vi "Amaster.vi"(8 "ErrorIn":errorcluster, 11 "AQueuesIn":T1) -> (0 "ErrorOut":errorcluster, 3 "AQueuesOut":T1)   [LabVIEW 2019]
uses:
  utilities/AQueues.ctl
  AmasterVIs/ACommand.ctl
  analyzeAccelerationDataVIs/AccelerationDataFrames.ctl
  analyzeAccelerationDataVIs/AnalyzedVibrationsData.ctl
  analyzeAccelerationDataVIs/calculateFaultIndicatorsVIs/FaultDetections.ctl
  analyzeAccelerationDataVIs/calculateFaultIndicatorsVIs/ParameterFaultDetection.ctl
  analyzeAccelerationDataVIs/calculateFaultIndicatorsVIs/FaultParameter.ctl
  analyzeAccelerationDataVIs/calculateFaultIndicatorsVIs/FrequencyFaultDetection.ctl
  analyzeAccelerationDataVIs/calculateFaultIndicatorsVIs/OrdersFaultDetection.ctl
  TDMSmanagerVIs/TDMSAnalyzerData.ctl
  TDMSmanagerVIs/TDMSAnalyzerDataType.ctl
  <vilib>/Platform/TimedLoop/XDataNode/timing_clust.ctl
  <vilib>/Platform/TimedLoop/XDataNode/nitl_modes.ctl
  <vilib>/Platform/TimedLoop/XDataNode/wakeup.ctl
  AmasterVIs/ACommandQueuesAction.ctl
  AmasterVIs/AThreads.ctl
  UIVIs/UIOutputFGVAction.ctl
  <vilib>/platform/TimedLoop/XDataNode/XDataNode.xnode
  <vilib>/Platform/TimedLoop/XDataNode/XDNodeRunTimeDep.lvlib
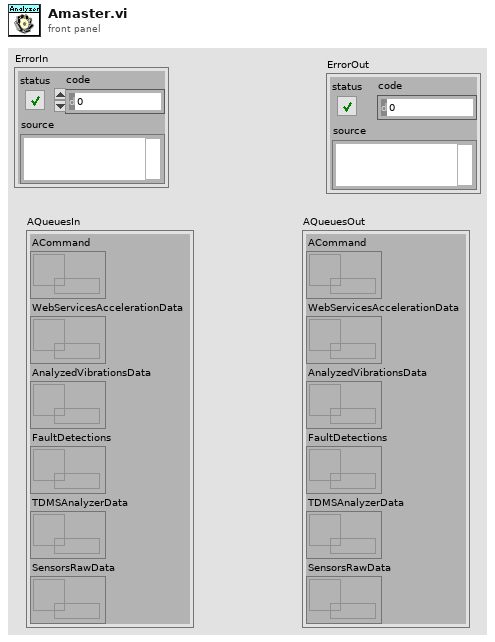
[diagram p1: front panel]
types:
  T1 = typedef "AQueues.ctl" = cluster{"ACommand":refnum<queue>, "WebServicesAccelerationData":refnum<queue>, "AnalyzedVibrationsData":refnum<queue>, "FaultDetections":refnum<queue>, "TDMSAnalyzerData":refnum<queue>, "SensorsRawData":refnum<queue>}
  T2 = typedef "XDNodeRunTimeDep.lvlib/timing_clust.ctl" = cluster{"Expected End [f-1]":u64, "Actual End [f-1]":u64, "Finished Late? [f-1]":bool, "Expected End [i-1]":u64, "Actual End [i-1]":u64, "Finished Late? [i-1]":bool, "Expected Start [i]":u64, "Actual Start [i]":u64, "Expected Start [f]":u64, "Actual Start [f]":u64, "Source Name":string, "Structure Name":string, "Period":i64, "Deadline":i64, "Offset":i64, "Start":i64, "Priority":i32, "Timeout":i32, "Mode":T3, "Wakeup Reason":T4, "Error":errorcluster, "Source Type":string, "Secondary Source Type":string, "Global End Time":u64, "Global Start Time":u64, "Frame Duration":u64, "Iteration Duration":u64, "Assigned CPU":i32, "I/O Scan Engine Mode":u32}
  T3 = typedef "XDNodeRunTimeDep.lvlib/nitl_modes.ctl" = enum32{"No Change", "Process missed periods, maintain original phase", "Discard missed periods, maintain original phase", "Process missed periods, ignore original phase", "Discard missed periods, ignore original phase"}
  T4 = typedef "XDNodeRunTimeDep.lvlib/wakeup.ctl" = enum32{"Normal", "Aborted", "Asynchronous wakeup", "Timing source error", "Timed loop error", "Timeout"}
  T5 = typedef "ACommandQueuesAction.ctl" = enum16{"Initialize", "Set", "Get", "ReleaseAll"}
  T6 = typedef "UIOutputFGVAction.ctl" = enum16{"Read", "Write", "CheckUpdate"}
  T7 = typedef "ACommand.ctl" = enum16{"None", "Start", "Stop", "Restart", "SendFilesData", "DeleteAllData"}
  T8 = typedef "AThreads.ctl" = enum16{"UI", "analyzeAccelerationData", "aquireAccelerationData", "communicateWebServices", "TDMSmanager", "aquireTachoSignal"}
  T9 = typedef "AnalyzerSettings.ctl" = cluster{"Create NS Timeout Code":i32, "Destroy NS Timeout Code":i32, "All threads":T8[], "AnalysisSettings":T10}
  T10 = typedef "AnalysisSettings.ctl" = cluster{"Fault Thresholds":T11, "Analysis series name":string, "Save data analysis?":bool, "Band size":i32, "OrderAnalysis?":bool, "Accelerometer":T13, "fs [Hz]":dbl, "Pulse per revolution":u16}
  T11 = typedef "Thresholds.ctl" = cluster{"Parameters labels":T12[], "Parameters thresholds":dbl[], "Freqs and thresholds":dbl[][], "Orders and thresholds":dbl[][]}
  T12 = typedef "FaultParameter.ctl" = enum16{"Kurtosis", "RMS", "Crest factor"}
  T13 = typedef "Accelerometer.ctl" = enum16{"None", "MPU6050", "MMA7351"}
  T14 = typedef "UIOutput.ctl" = cluster{"Aquiring data":bool, "AnalyzerError":errorcluster, "FIFO overflow":bool, "Analyzing data":bool}
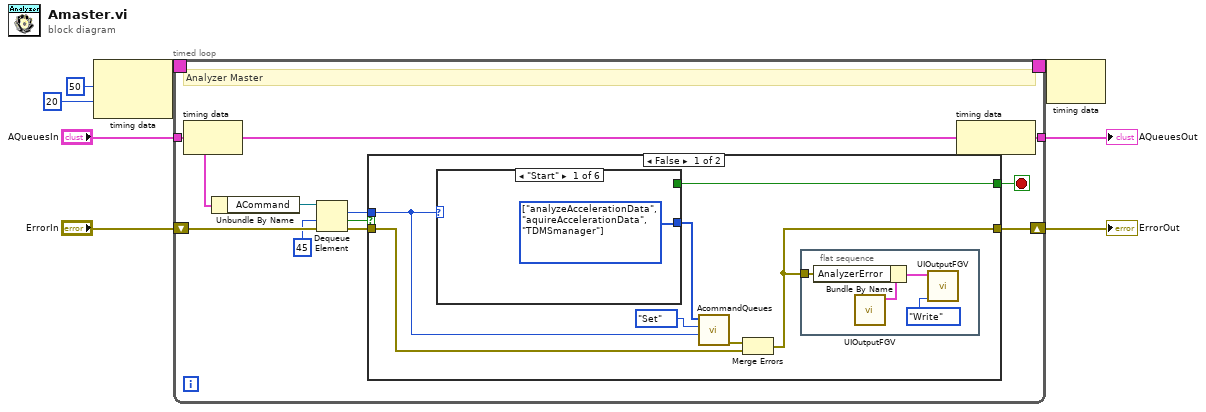
[diagram p0: block diagram]
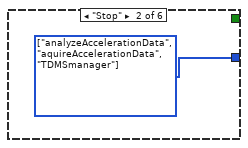
[diagram p2: hidden frame]
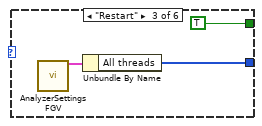
[diagram p3: hidden frame]
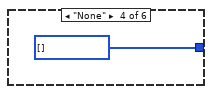
[diagram p4: hidden frame]
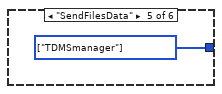
[diagram p5: hidden frame]
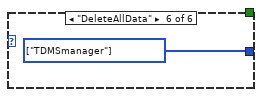
[diagram p6: hidden frame]
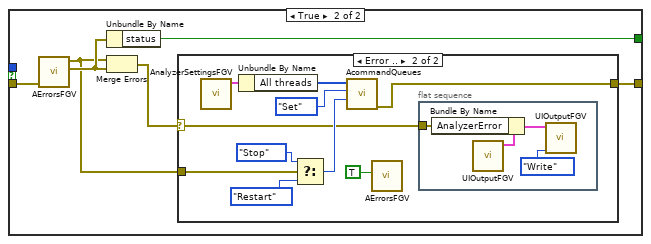
[diagram p7: hidden frame]
diagram:
  n1 = node-c288(i64 50 ("Period"), 20 ("Priority")) -> (w4:T2)
  n2 = timed-loop {
    tunnel: "AQueuesIn" -> [w11]
    shift-right: [w9] -> w7
    shift-left: "ErrorIn" -> [w16]
    tunnel: [w11] -> w5
    timing: w4 -> [_]
    timing-out: [_] -> w3
    stop <- w10 stop-if-true
    # "Analyzer Master"
    n3 = node-c288() -> ()  [unwired: 1 in, 1 out]
    n4 = Unbundle By Name(w11) -> ("ACommand"=w17:refnum<queue>)
    n5 = Dequeue Element(queue=w17, timeout in ms (-1)=45, error in (no error)=w16) -> (element=w12:T7, timed out?=w14:bool, error out=w13:errorcluster)  [unwired: 1 out]
    n6 = case shown="False" w14 {
      tunnel: w13 -> [w21 w41]
      tunnel: [w20 w44] -> w9
      tunnel: [w26 w43] -> w10
      tunnel: w12 -> [w23 _]
      frame False {
        n7 = case shown="\"Start\"" w23 {
          tunnel: [w31 w32 w33 w36 w37 w38] -> w25
          tunnel: [_ _ TRUE _ _ _] -> w26
          frame "Start" {
            w31 = T8[] [enum."analyzeAccelerationData", enum."aquireAccelerationData", enum."TDMSmanager"] items=["UI", "analyzeAccelerationData", "aquireAccelerationData", "communicateWebServices", "TDMSmanager", "aquireTachoSignal"] ("AThreads")
          }
          frame "Stop" {
            w32 = T8[] [enum."analyzeAccelerationData", enum."aquireAccelerationData", enum."TDMSmanager"] items=["UI", "analyzeAccelerationData", "aquireAccelerationData", "communicateWebServices", "TDMSmanager", "aquireTachoSignal"] ("AThreads")
          }
          frame "Restart" {
            n8 = call "AnalyzerSettingsFGV.vi"() -> ("GlobalSettingsOut"=w34:T9)  [unwired: 11 in]
            n9 = Unbundle By Name(w34) -> ("All threads"=w33:T8[])
          }
          frame "None" {
            w36 = T8[] [] items=["UI", "analyzeAccelerationData", "aquireAccelerationData", "communicateWebServices", "TDMSmanager", "aquireTachoSignal"] ("AThreads")
          }
          frame "SendFilesData" {
            w37 = T8[] [enum."TDMSmanager"] items=["UI", "analyzeAccelerationData", "aquireAccelerationData", "communicateWebServices", "TDMSmanager", "aquireTachoSignal"] ("AThreads")
          }
          frame "DeleteAllData" {
            w38 = T8[] [enum."TDMSmanager"] items=["UI", "analyzeAccelerationData", "aquireAccelerationData", "communicateWebServices", "TDMSmanager", "aquireTachoSignal"] ("AThreads")
          }
        }
        n10 = call "AcommandQueues.vi"("ACommandIn"=w23, "ACommandQueuesAction"=ACommandQueuesAction."Set", "AThreads"=w25) -> ("ErrorOut"=w22:errorcluster)  [unwired: 7 in, 1 out]
        n11 = Merge Errors(w22, w21) -> (w20:errorcluster)
        n12 = flat-sequence {
          tunnel: w20 -> [w29]
          frame #0 {
            n13 = call "UIOutputFGV.vi"() -> ("UIOutputOut"=w30:T14)  [unwired: 10 in, 1 out]
            n14 = Bundle By Name(cluster=w30, "AnalyzerError"=w29) -> (w28:T14)
            n15 = call "UIOutputFGV.vi"("FGVAction (Read)"=UIOutputFGVAction."Write", "UIOutputIn"=w28) -> ()  [unwired: 8 in, 2 out]
          }
        }
      }
      frame True {
        n16 = call "AErrorsFGV.vi"("CriticalErrorIn"=w41) -> ("GetCriticalError"=w40:errorcluster, "GetInternalError"=w39:errorcluster)  [unwired: 7 in, 2 out]
        n17 = Unbundle By Name(w40) -> ("status"=w43:bool)
        n18 = Merge Errors(w39, w40) -> (w42:errorcluster)
        n19 = case shown="Error .." w42 {
          selector: w42 -> [w45 w47]
          tunnel: [w45 w48] -> w44
          tunnel: w39 -> [_ w49]
          frame No Error {
          }
          frame Error {
            n20 = call "AnalyzerSettingsFGV.vi"() -> ("GlobalSettingsOut"=w55:T9)  [unwired: 11 in]
            n21 = Unbundle By Name(w55) -> ("All threads"=w54:T8[])
            n22 = Select(t=ACommand."Stop" ("ACommandIn"), s=w49, f=ACommand."Restart") -> (s? t:f=w50:T7)
            n23 = call "AcommandQueues.vi"("ACommandIn"=w50, "ACommandQueuesAction"=ACommandQueuesAction."Set", "AThreads"=w54) -> ("ErrorOut"=w48:errorcluster)  [unwired: 7 in, 1 out]
            n24 = call "AErrorsFGV.vi"("Reset?"=TRUE) -> ()  [unwired: 7 in, 4 out]
            n25 = flat-sequence {
              tunnel: [w56] -> _
              tunnel: w47 -> [w56]
              frame #0 {
                n26 = call "UIOutputFGV.vi"() -> ("UIOutputOut"=w59:T14)  [unwired: 10 in, 1 out]
                n27 = Bundle By Name(cluster=w59, "AnalyzerError"=w56) -> (w58:T14)
                n28 = call "UIOutputFGV.vi"("FGVAction (Read)"=UIOutputFGVAction."Write", "UIOutputIn"=w58) -> ()  [unwired: 8 in, 2 out]
              }
            }
          }
        }
      }
    }
    n29 = node-c288() -> ()  [unwired: 1 in, 1 out]
  }
  "ErrorOut" <- w7
  "AQueuesOut" <- w5
  n30 = node-c288(w3) -> ()  [unwired: 1 out]
